vi "Set Next Turn.vi"(0 "comm interface in":refnum<class "Pixy Com.lvclass">, 5 "next turn angle":i16 min=-90 max=90 step=1, 11 "error in":errorcluster) -> (4 "comm interface out":refnum<class "Pixy Com.lvclass">, 15 "error out":errorcluster)   [LabVIEW 2018, in "Pixy2.lvlib"]
doc: "Sets the next turn angle for the Line Tracking algorithm. This overrides the default turn angle for the next intersection."
uses:
  Pixy2.lvlib
  Interface/Pixy Com.lvclass
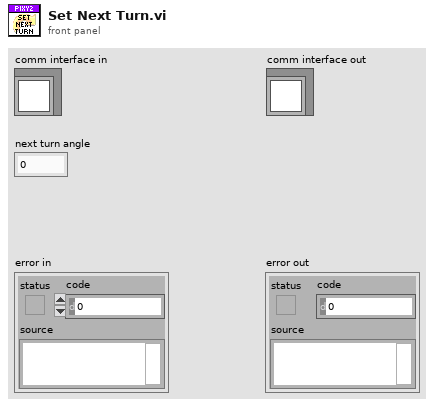
[diagram p1: front panel]
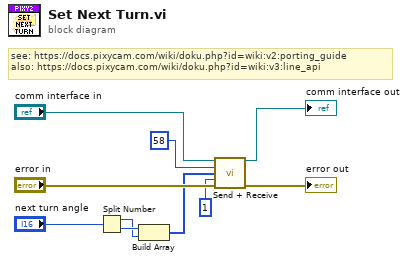
[diagram p0: block diagram]
diagram:
  # "see: https://docs.pixycam.com/wiki/doku.php?id=wiki:v2:porting_guide\nalso: https://docs.pixycam.com/wiki/doku.php?id=wiki:v3:line_api"
  n1 = Split Number(x="next turn angle") -> (hi(x)=w8:u8, lo(x)=w9:u8)
  n2 = Build Array(w9, w8) -> (w2:u8[])
  n3 = call "Send + Receive.vi"("comm interface in"="comm interface in", "type"=u8 58, "payload"=w2, "expected response"=u8 1 ("expected type"), "error in"="error in") -> ("comm interface out"=→"comm interface out":refnum<class "Pixy Com.lvclass">, "error out"=→"error out":errorcluster)  [unwired: 8 in, 1 out]
